vi "GitCommit.vi"(4 "CommitAllAdded":bool, 5 "Date":string, 6 "Allow Empty Commit?":bool, 7 "Author":string, 8 "error in (no error)":errorcluster, 9 "File":path=path "", 10 "Commit Message":string, 11 "Git exec":string="git") -> (0 "error out":errorcluster, 1 "File out":path, 2 "Response":string, 3 "Git exec out":string="git")   [LabVIEW 2013]
uses:
  GitCmd.vi
  <vilib>/dlg_ctls.llb/Space Constant.vi
  <vilib>/Utility/error.llb/General Error Handler.vi
  GitUtils/PathtoDirPath.vi
  <vilib>/Platform/system.llb/System Exec.vi
  <vilib>/Utility/error.llb/Error Cluster From Error Code.vi
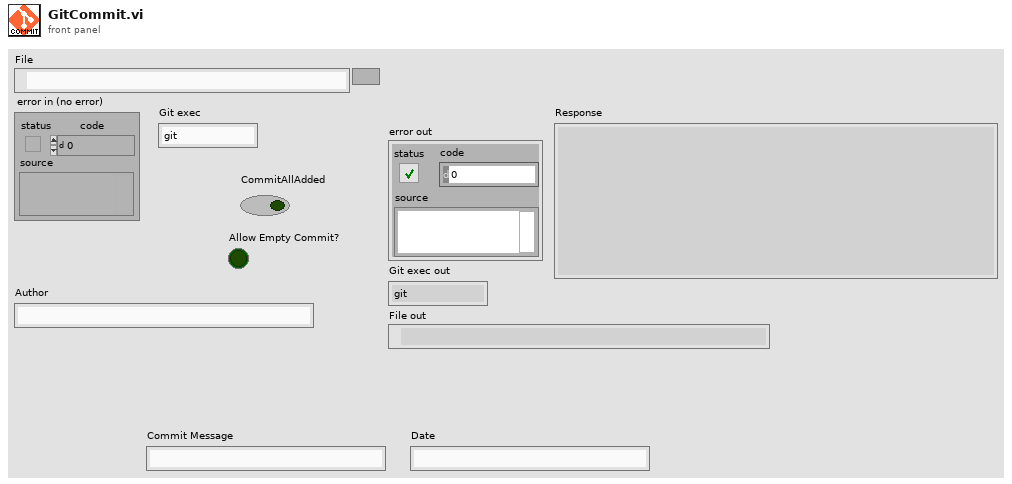
[diagram p1: front panel]
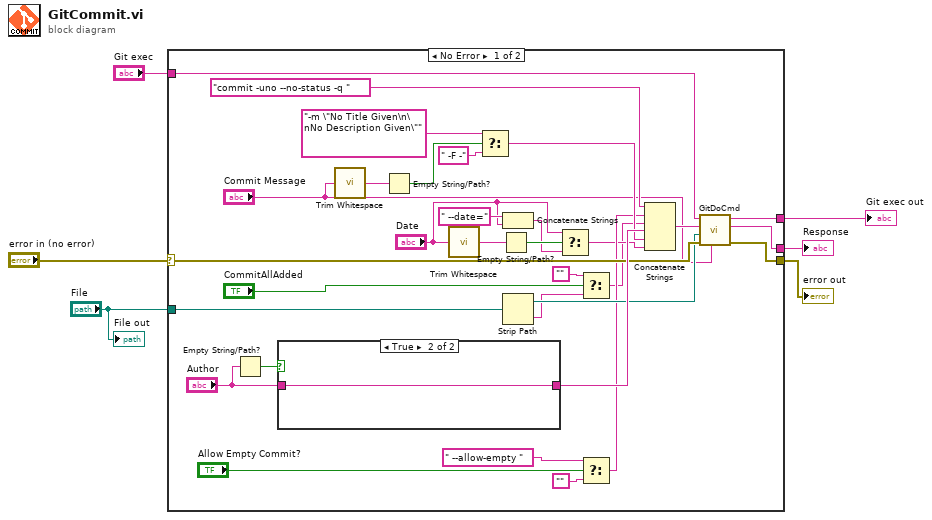
[diagram p0: block diagram]
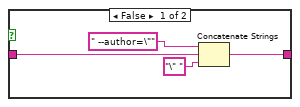
[diagram p2: hidden frame]
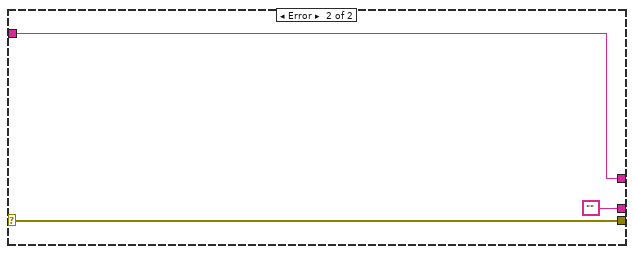
[diagram p3: hidden frame]
diagram:
  n1 = case shown="No Error" "error in (no error)" {
    selector: "error in (no error)" -> [w28 w45]
    tunnel: "Git exec" -> [w32 w44]
    tunnel: "File" -> [w37 _]
    tunnel: [w30 ""] -> w3
    tunnel: [w29 w45] -> w2
    tunnel: [w31 w44] -> w1
    frame No Error {
      n2 = Empty String/Path?(string/path="Author") -> (empty?=w36:bool)
      n3 = case shown="True" w36 {
        tunnel: [w41 w43] -> w34
        tunnel: "Author" -> [w42 w43]
        frame False {
          n4 = Concatenate Strings(" --author=\"" ("string"), w42, "\" " ("string")) -> (w41:string)
        }
        frame True {
        }
      }
      n5 = call <vilib>:"Trim Whitespace.vi"("string"="Commit Message") -> ("trimmed string"=w21:string)  [unwired: 1 in]
      n6 = Empty String/Path?(string/path=w21) -> (empty?=w26:bool)
      n7 = call <vilib>:"Trim Whitespace.vi"("string"="Date") -> ("trimmed string"=w16:string)  [unwired: 1 in]
      n8 = Select(t="-m \"No Title Given\n\nNo Description Given\"", s=w26, f=" -F -" ("string")) -> (s? t:f=w24:string)
      n9 = Empty String/Path?(string/path=w16) -> (empty?=w15:bool)
      n10 = Concatenate Strings(" --date=" ("string"), "Date") -> (w12:string)
      n11 = Strip Path(path=w37) -> (stripped path=w27:path, name=w9:string)
      n12 = Select(t="Date", s=w15, f=w12) -> (s? t:f=w11:string)
      n13 = Select(t="", s="CommitAllAdded", f=w9) -> (s? t:f=w8:string)
      n14 = Select(t=" --allow-empty ", s="Allow Empty Commit?", f="") -> (s? t:f=w17:string)
      n15 = Concatenate Strings("commit -uno --no-status -q " ("string"), w17, w8, w34, w24, w11) -> (w33:string)
      n16 = call "GitDoCmd.vi"("standard input"="Commit Message", "error in (no error)"=w28, "Working Path"=w27, "Git command"=w33, "Git exec"=w32) -> ("error out"=w29:errorcluster, "Returned stdout"=w30:string, "Git exec out"=w31:string)  [unwired: 2 in, 1 out]
    }
    frame Error {
    }
  }
  "Response" <- w3
  "error out" <- w2
  "Git exec out" <- w1
  "File out" <- "File"
